vi "RF Rec Read Debug Signals.vi"(2 "Debug CLIP Resources":T2={"Hard Error"="PXIe-6592R IO Socket v1\\uPort0_HardError", "Soft Error"="PXIe-6592R IO Socket v1\\uPort0_HardError", "Lane Up"="PXIe-6592R IO Socket v1\\uPort0_HardError", "Channel Up"="PXIe-6592R IO Socket v1\\uPort0_HardError", "Sys Reset"="PXIe-6592R IO Socket v1\\uPort0_HardError"}) -> (4 "port debug info":T1)   [LabVIEW 2018]
doc: "Reads debug signals from the CLIP.\n\n<B>Input Parameters</B>\n\n<B>Debug CLIP Resources</B> specifies the CLIP Resources used for debug signals.\n\n<B>Debug CLIP Resources.Hard Error</B> specifies the CLIP Resource used to indicate a Hard Error.\n\n<B>Debug CLIP Resources.Soft Error</B> specifies the CLIP Resource used to indicate a Soft Error.\n\n<B>Debug CLIP Resources.Lane Up</B> specifies the CLIP Resource used to indicate whether the Lane is Up.\n\n<B>Debug CLIP Resources.Channel Up</B> specifies the CLIP Resource used to indicate whether the Channel is Up.\n\n<B>Debug CLIP Resources.Sys Reset</B> specifies the CLIP Resource used to indicate if the System is in Reset.\n\n<B>Output Parameters</B>\n\n<B>Debug Info</B> contains debug information read from the CLIP.\n\n<B>Debug Info.Hard Error</B> indicates whether a Hard Error has occurred.\n\n<B>Debug Info.Soft Error</B> indicates whether a Soft Error has occurred.\n\n<B>Debug Info.Lane Up</B> indicates whether the Lane is Up.\n\n<B>Debug Info.Channel Up</B> indicates whether the Channel is Up.\n\n<B>Debug Info.Sys Reset</B> indicates whether the System is in Reset."
uses:
  RF Rec Port Debug Info.ctl
  <vilib>/rvi/eio/common/nirviEmuTemplateMethod_errors.vi
  <vilib>/eio/EIONode/EIONode.xnode
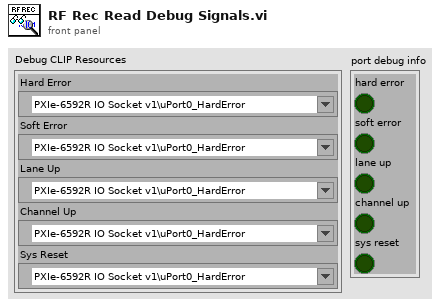
[diagram p1: front panel]
types:
  T1 = typedef "RF Rec Port Debug Info.ctl" = cluster{"hard error":bool, "soft error":bool, "lane up":bool, "channel up":bool, "sys reset":bool}
  T2 = cluster{"Hard Error":refnum<k21>, "Soft Error":refnum<k21>, "Lane Up":refnum<k21>, "Channel Up":refnum<k21>, "Sys Reset":refnum<k21>}
  T3 = cluster{"Hard Error":bool, "Soft Error":bool, "Lane Up":bool, "Channel Up":bool, "Sys Reset":bool}
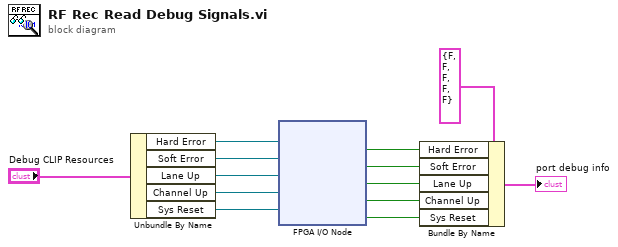
[diagram p0: block diagram]
diagram:
  n1 = Unbundle By Name("Debug CLIP Resources") -> ("Hard Error"=w12:refnum<k21>, "Soft Error"=w11:refnum<k21>, "Lane Up"=w10:refnum<k21>, "Channel Up"=w9:refnum<k21>, "Sys Reset"=w8:refnum<k21>)
  n2 = xnode "FPGA I/O Node"("FPGA I/O In"=w12, "FPGA I/O In"=w11, "FPGA I/O In"=w10, "FPGA I/O In"=w9, "FPGA I/O In"=w8) -> ("I/O Item"=w7:bool, "I/O Item"=w6:bool, "I/O Item"=w5:bool, "I/O Item"=w4:bool, "I/O Item"=w3:bool)  [unwired: 5 out]
  n3 = Bundle By Name(cluster=T3 {"Hard Error"=FALSE, "Soft Error"=FALSE, "Lane Up"=FALSE, "Channel Up"=FALSE, "Sys Reset"=FALSE} ("Debug Values"), "Hard Error"=w7, "Soft Error"=w6, "Lane Up"=w5, "Channel Up"=w4, "Sys Reset"=w3) -> (→"port debug info":T3)
